vi "Main.vi"() -> ()   [LabVIEW 2015]
doc: "This template is for the Queued Message Handler design pattern.\n\nThe Event Handling Loop generates messages based on user interface actions.\n\nThe Message Handling Loop processes messages generated by the Event Handling Loop, or by other messages. The messages are string values, so new messages can be added easily to the Message Cases case structure in the Message Handling Loop. Each message cluster can also provide an optional value for Message Data, which is a variant that can be converted to whatever message-specific data is required."
uses:
  Custom Controls/config.ctl
  <vilib>/MakerHub/LINX/Private/Type Defs/LINX Ref.ctl
  <vilib>/MakerHub/LINX/Private/Type Defs/Platform.ctl
  <vilib>/MakerHub/LINX/Private/Type Defs/Interface.ctl
  <vilib>/MakerHub/LINX/Private/Device/Type Defs/LINX Device Config.ctl
  <vilib>/MakerHub/LINX/Private/Device/Type Defs/TCP Config.ctl
  <vilib>/MakerHub/LINX/Private/Device/Type Defs/Channels.ctl
  <vilib>/MakerHub/LINX/Public/Peripherals/PWM/PWM Set Duty Cycle 1 Chan.vi
  <vilib>/MakerHub/LINX/Public/Peripherals/Digital/Digital Write 1 Chan.vi
  <vilib>/MakerHub/LINX/Public/Peripherals/Analog/Analog Read 1 Chan.vi
  <vilib>/MakerHub/LINX/Public/Peripherals/Digital/Digital Write N Chans.vi
  <vilib>/MakerHub/LINX/Public/Peripherals/Analog/Analog Read N Chans.vi
  <vilib>/MakerHub/LINX/Private/Local IO/LinxDigitalWrite.vi
  <vilib>/MakerHub/LINX/Public/Utilities/Check Channel.vi
  <vilib>/MakerHub/LINX/Private/Local IO/LinxAnalogRead.vi
  support/Message Queue/Enqueue Message (Single).vi
  <vilib>/Utility/error.llb/Error Cluster From Error Code.vi
  <vilib>/MakerHub/LINX/Public/Utilities/Open Serial.vi
  <vilib>/MakerHub/LINX/Public/Peripherals/PWM/PWM Set Duty Cycle N Chans.vi
  <vilib>/MakerHub/LINX/Private/Utilties/Generate Error.vi
  <vilib>/MakerHub/LINX/Public/Sensors/Motion/Servo/Servo Open One Channel.vi
  <vilib>/MakerHub/LINX/Public/Sensors/Motion/Servo/Servo Set Pulse Width One Channel.vi
  <vilib>/MakerHub/LINX/Public/Sensors/Motion/Servo/Servo Close One Channel.vi
  <vilib>/ErrorRing/Error Ring.xnode
  support/Message Queue/Message Queue.lvlib
  support/User Event - Stop/User Event - Stop.lvlib
  <vilib>/MakerHub/LINX/LMH-LINX.lvlib
  <vilib>/MakerHub/LINX/Public/Sensors/Pmods/GPS/PmodGPS.lvlib
  <vilib>/MakerHub/LINX/Public/Sensors/Motion/Servo/Servo.lvlib
  <vilib>/MakerHub/LINX/Private/Device/Device.lvlib
panel:
  out "Bearing Diff. (deg)":dbl
  out "Actuator Duty Cycle":cluster{"Active":dbl, "Rest":dbl}(graph)
  out "Active Actuator Time (s)":dbl
  out "Required Delay":dbl
  in  "Actuator Channels":T1={"PWM Channel"=9, "Extend Channel"=11, "Retract Channel"=13}
  out "error (out)":errorcluster
  out "Current Bearing (deg)":dbl caption="Numeric"
  out "\"deg\"":string="               deg" caption="String"
  out "Compass":cluster{dbl, dbl}(knob)={0.0, 64.08711650949901} scale=0.0..360.0
  out "Action Feed":string
  out "\"mph\"":string="               mph" caption="String"
  out "Speed Dec":dbl caption="Numeric" format="%#_3g"
  out "\"rpm\"":string="                  rpm" caption="String"
  out "RPM Dec":dbl caption="Numeric"
  out "Steering Angle":dbl(knob) scale=-30.0..30.0
  out "Fuel Meter":dbl(knob) scale=0.0..100.0
  out "Waypoints remaining:":i32 caption="Numeric"
  out "En Route to Waypoint:":i32 caption="Numeric"
  out "Progress Bar":u8(slide) scale=0.0..100.0
  out "Speed Gauge":dbl(knob) scale=0.0..25.0
  out "RPM Gauge":dbl(knob) scale=0.0..7.0
  out "Radio Signal Strength":dbl[](graph)
  out "Steering Angle":T2(graph)
  in  "VISA resource":refnum<visa-resource-name>="COM6"
  out "GPS Data":T3
  in  "WebBrowser":refnum<k7>(container)
  in  "EARTHLib.IApplicationGE 2":refnum<k7>
  out "Init. Panel":cluster{"Boolean":bool, "String":string}[][](array[cluster])
  in  "Abort":bool
  in  "Config":T4
  in  "Open Path":bool caption="Open"
  in  "Start":bool
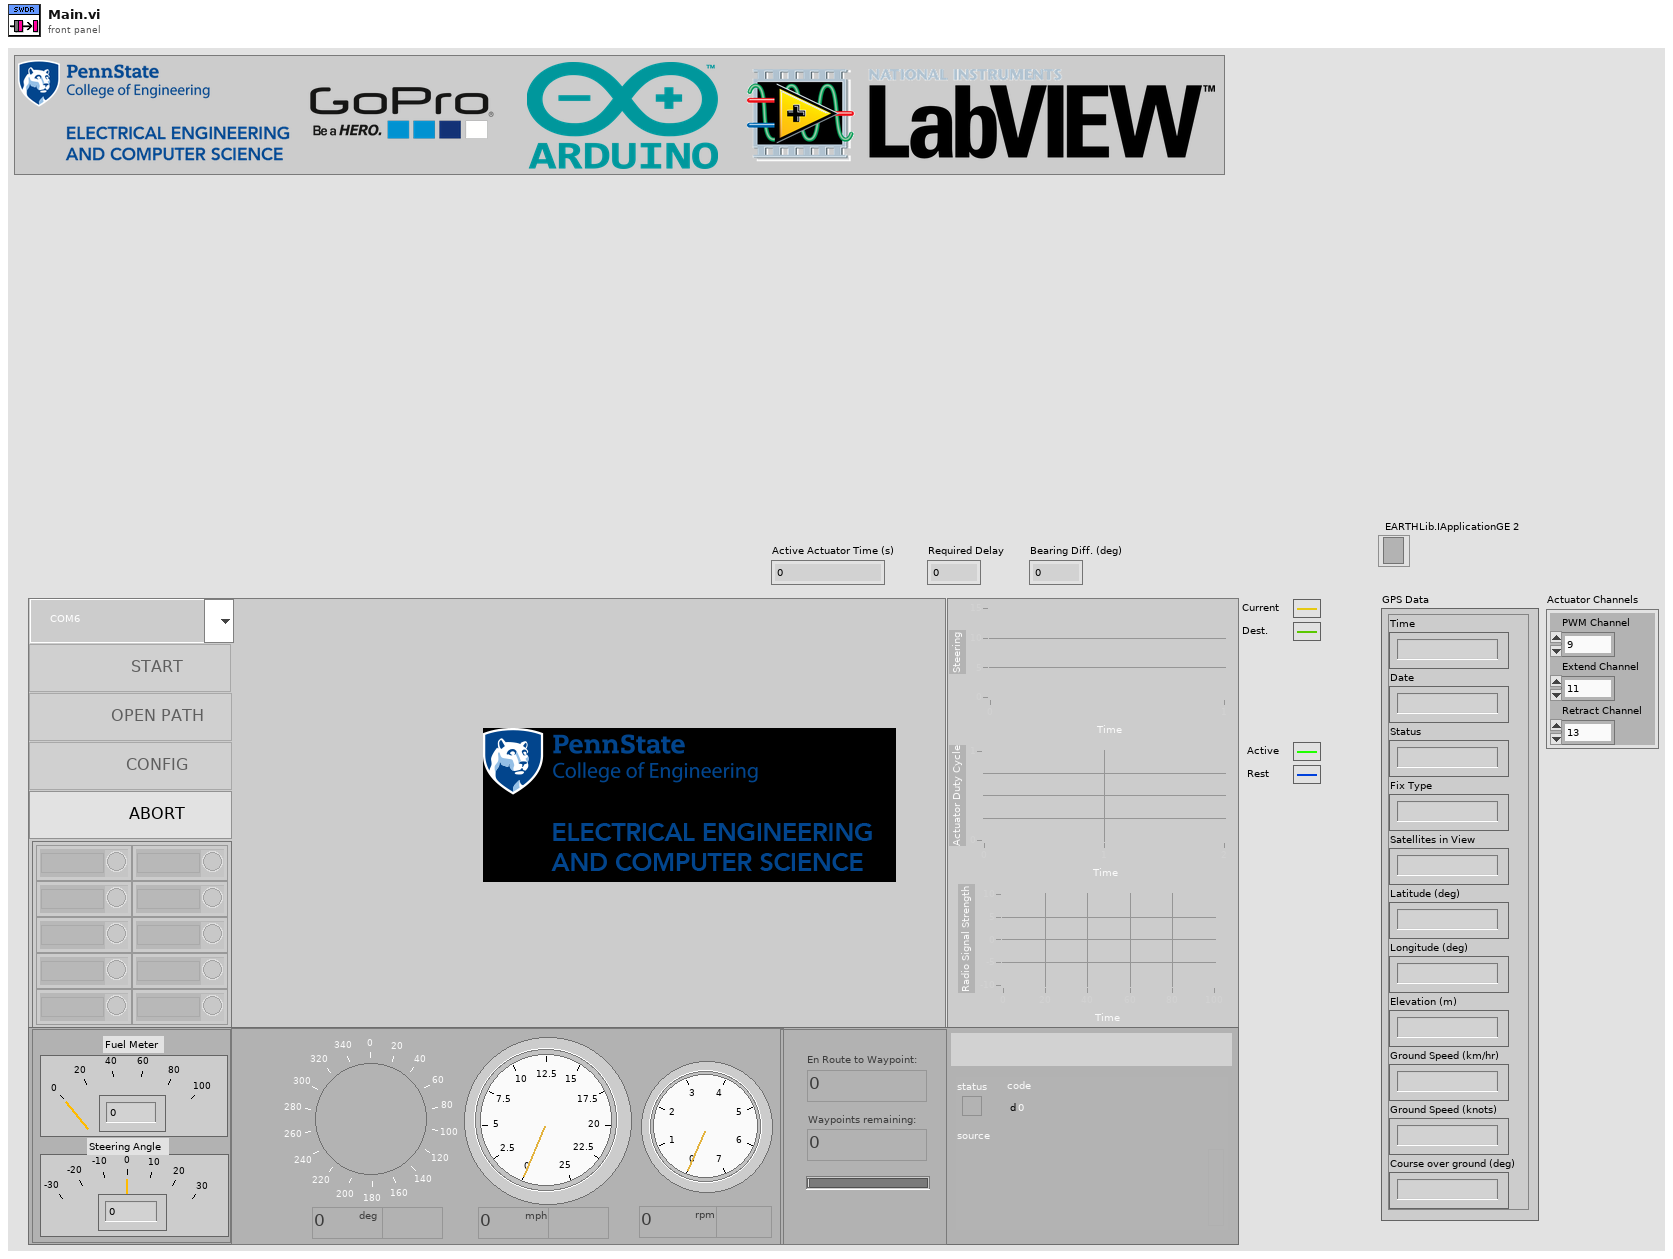
[diagram p1: front panel]
types:
  T1 = cluster{"PWM Channel":u8, "Extend Channel":u8, "Retract Channel":u8}
  T2 = cluster{"Current Bearing (deg)":dbl, "Bearing to Waypoint (deg)":dbl}
  T3 = cluster{"Time":string, "Date":string, "Status":string, "Fix Type":string, "Satellites in View":string, "Latitude (deg)":string, "Longitude (deg)":string, "Elevation (m)":string, "Ground Speed (km/hr)":string, "Ground Speed (knots)":string, "Course over ground (deg)":string}
  T4 = typedef "config.ctl" = bool
  T5 = typedef "LMH-LINX.lvlib/LINX Ref.ctl" = cluster{"IO":T6, "Interface":T7, "LINX Device Config":T8}
  T6 = typedef "LMH-LINX.lvlib/Platform.ctl" = enum16{"Remote", "Local"}
  T7 = typedef "LMH-LINX.lvlib/Interface.ctl" = enum16{"Serial", "TCP"}
  T8 = typedef "LMH-LINX.lvlib/Device.lvlib/LINX Device Config.ctl" = cluster{"Interface":T7, "COM Port":refnum<visa-resource-name>, "TCP Configuration":T9, "Device Family":u8, "Device ID":u8, "Device Name":string, "TCP Ref":refnum<k5>, "Channels":T10}
  T9 = typedef "LMH-LINX.lvlib/Device.lvlib/TCP Config.ctl" = cluster{"IP Address":string, "Port":u16}
  T10 = typedef "LMH-LINX.lvlib/Channels.ctl" = cluster{"DI":u8[], "DO":u8[], "AI":u8[], "AO":u8[], "PWM":u8[], "QE":u8[], "UART":u8[], "I2C 2":u8[], "SPI":u8[], "CAN":u8[], "Servo":u8[], "AI Ref (V)":dbl, "AI Resolution (Bits)":u8, "AO Ref (V)":dbl, "AO Resolution (Bits)":u8}
  T11 = cluster{"Waypoint Array":cluster{"Latitude":dbl, "Longitude":dbl}[], "GPS Data":cluster{"Time":string, "Date":string, "Status":string, "Fix Type":string, "Satellites in View":string, "Latitude (deg)":string, "Longitude (deg)":string, "Elevation (m)":string, "Ground Speed (km/hr)":string, "Ground Speed (knots)":string, "Course over ground (deg)":string}, cluster{"Marker":string, "Path":string, "Markers Coordinates":string[][]}, "LINX Resource":T5, "Google Earth Ref":refnum<k7>, "Time":timestamp, "Waypoint Array Size":i32}
  T12 = typedef "Message Queue.lvlib/All Message Queues.ctl" = cluster{"UI":refnum<queue>}
  T13 = cluster{"Current Bearing":dbl, "Bearing to WP.":dbl}
  T14 = enum8{"Enabled", "Disabled", "Disabled and Grayed Out"}
  T15 = cluster{"Waypoint Array":cluster{"Latitude":dbl, "Longitude":dbl}[], "GPS Data":cluster{"Time":string, "Date":string, "Status":string, "Fix Type":string, "Satellites in View":string, "Latitude (deg)":string, "Longitude (deg)":string, "Elevation (m)":string, "Ground Speed (km/hr)":string, "Ground Speed (knots)":string, "Course over ground (deg)":string}, "Cluster":cluster{"Marker":string, "Path":string, "Markers Coordinates":string[][]}, "LINX Resource":T5, "Google Earth Ref":refnum<k7>, "Time":timestamp, "Waypoint Array Size":i32}
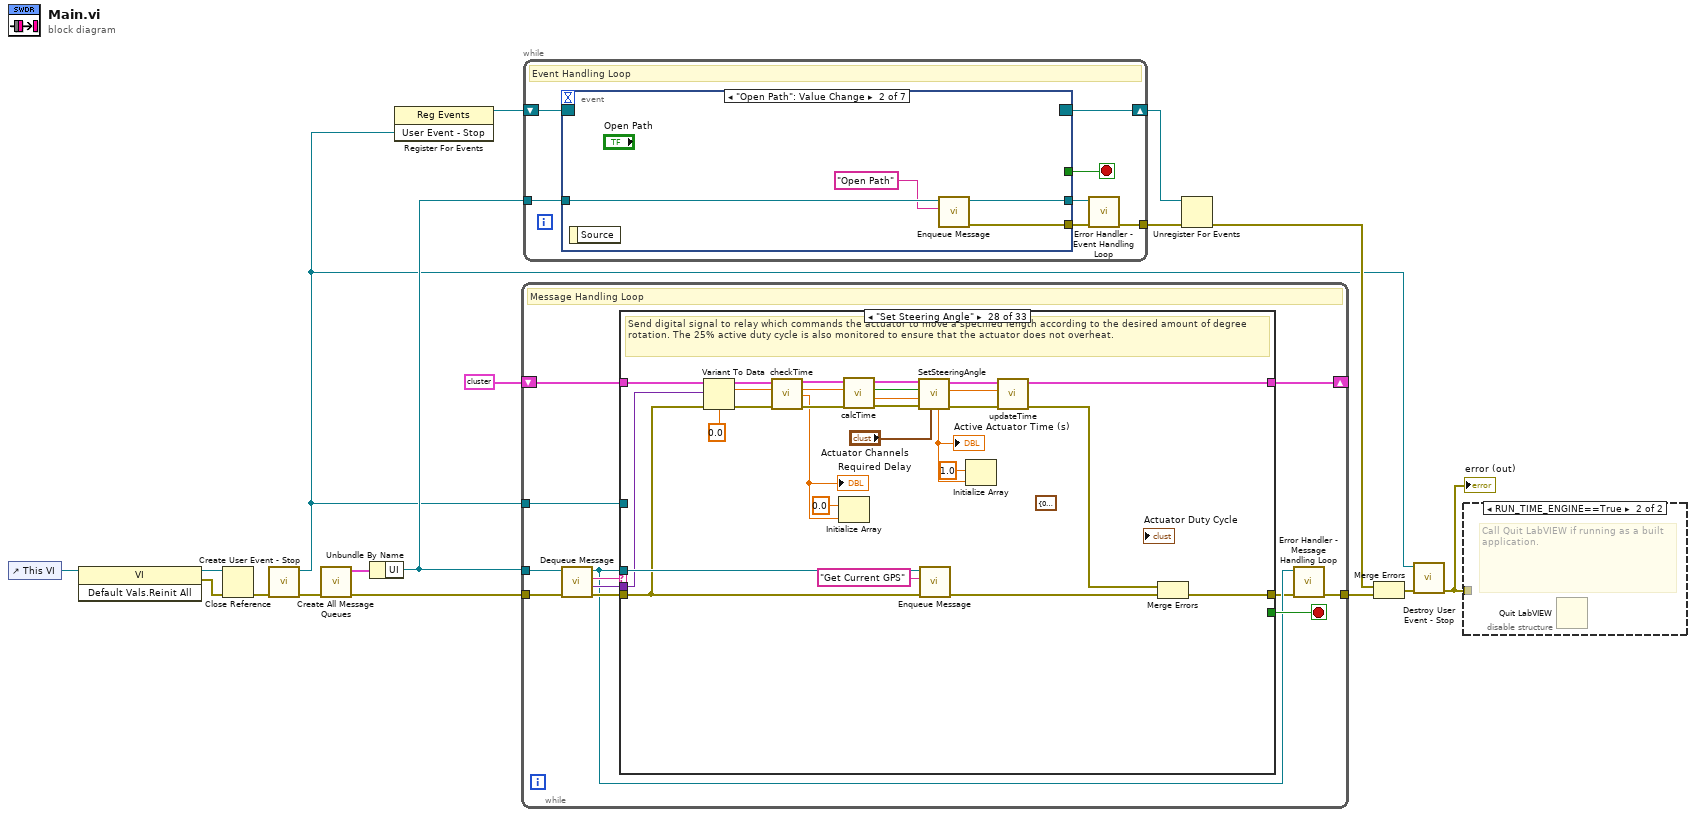
[diagram p0: block diagram]
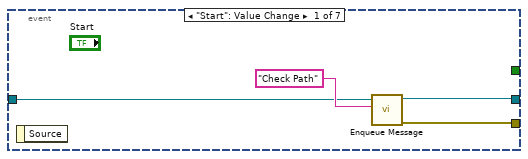
[diagram p3: hidden frame]
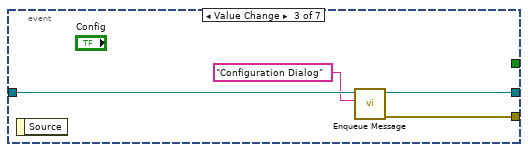
[diagram p4: hidden frame]
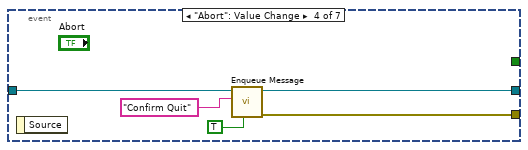
[diagram p5: hidden frame]
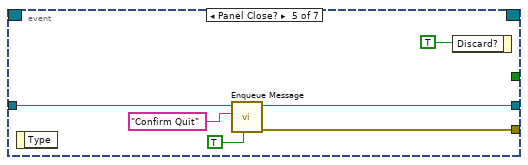
[diagram p6: hidden frame]
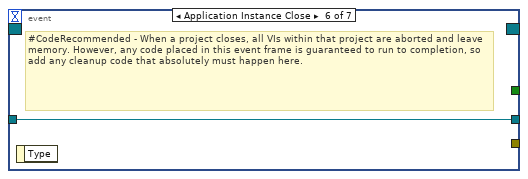
[diagram p7: hidden frame]
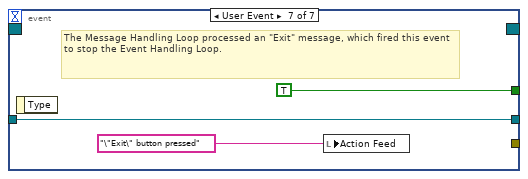
[diagram p8: hidden frame]
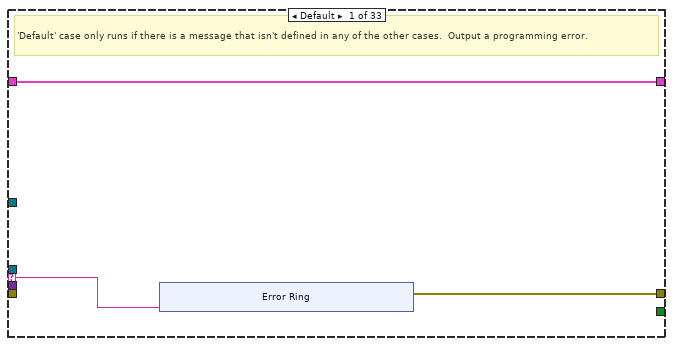
[diagram p9: hidden frame]
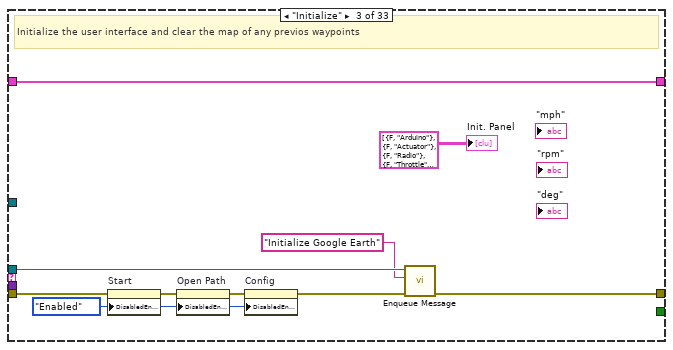
[diagram p11: hidden frame]
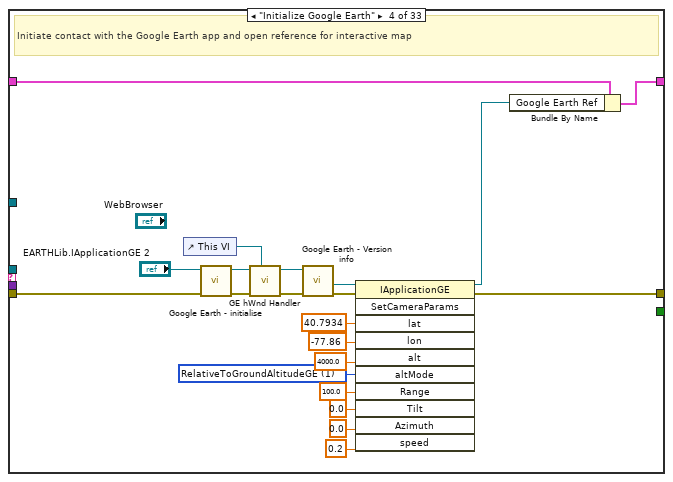
[diagram p12: hidden frame]
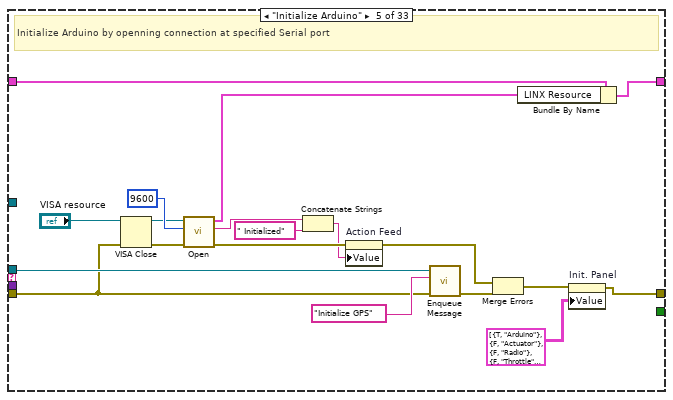
[diagram p13: hidden frame]
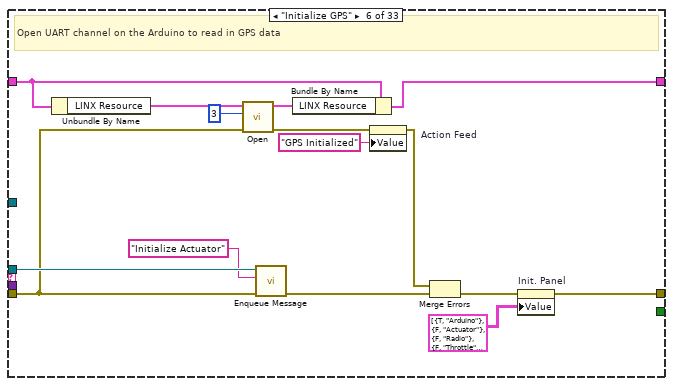
[diagram p14: hidden frame]
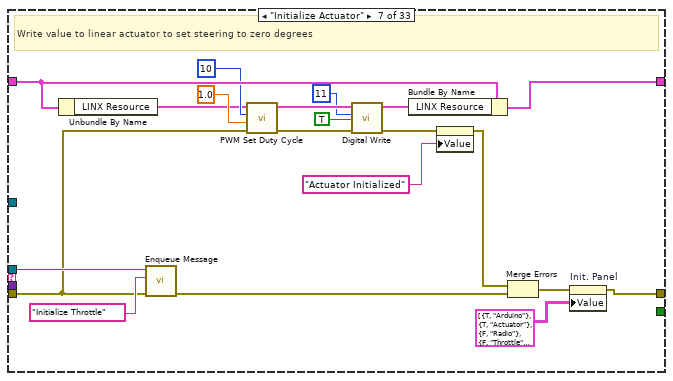
[diagram p15: hidden frame]
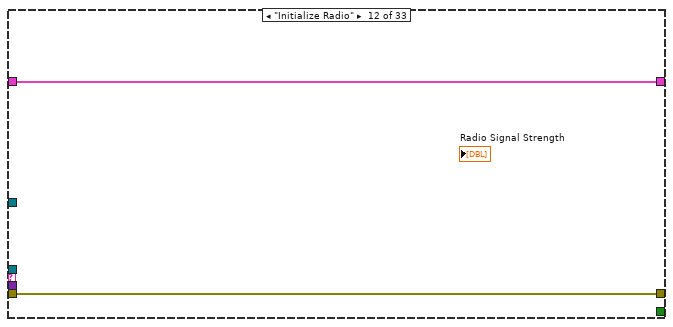
[diagram p20: hidden frame]
diagram:
  n1 = control-ref of="This VI"() -> (w7:refnum<vi>)
  n2 = invoke class="VI" method="Default Vals.Reinit All"(reference=w7) -> (reference out=w6:refnum<vi>, error out=w5:errorcluster)  [unwired: 2 in, 1 out]
  n3 = Close Reference(reference=w6, error in (no error)=w5) -> (error out=w4:errorcluster)
  n4 = call "Create User Event - Stop.vi"("error in (no error)"=w4) -> ("error out"=w14:errorcluster, "User Event - Stop"=w8:refnum<user-event>)  [unwired: 9 in]
  n5 = call "Create All Message Queues.vi"("error in (no error)"=w14) -> ("error out"=w3:errorcluster, "Message Queues out"=w17:T12)  [unwired: 9 in]
  n6 = Unbundle By Name(w17) -> ("UI"=w15:refnum<queue>)
  n7 = register-events(w8) -> (reference out=w9:refnum<event-registration>)  [unwired: 2 in, 1 out]
  n8 = while {
    tunnel: w15 -> [w23]
    tunnel: w8 -> [w28]
    tunnel: w3 -> [w27]
    tunnel: [w21] -> w16
    shift-right: [w18] -> _
    shift-left: T11 {"Waypoint Array"=[], "GPS Data"={"Time"="", "Date"="", "Status"="", "Fix Type"="", "Satellites in View"="", "Latitude (deg)"="", "Longitude (deg)"="", "Elevation (m)"="", "Ground Speed (km/hr)"="", "Ground Speed (knots)"="", "Course over ground (deg)"=""}, {"Marker"="", "Path"="", "Markers Coordinates"=[]}, "LINX Resource"={"IO"=enum."Remote", "Interface"=enum."Serial", "LINX Device Config"={"Interface"=enum."Serial", "COM Port"="", "TCP Configuration"={"IP Address"="", "Port"=0}, "Device Family"=0, "Device ID"=0, "Device Name"="", "TCP Ref"=refnum, "Channels"={"DI"=[], "DO"=[], "AI"=[], "AO"=[], "PWM"=[], "QE"=[], "UART"=[], "I2C 2"=[], "SPI"=[], "CAN"=[], "Servo"=[], "AI Ref (V)"=0.0, "AI Resolution (Bits)"=0, "AO Ref (V)"=0.0, "AO Resolution (Bits)"=0}}}, "Google Earth Ref"=refnum, "Time"=timestamp(0 s since 1904-01-01), "Waypoint Array Size"=0} -> [w19]
    stop <- w29 stop-if-true
    # "Message Handling Loop"
    n9 = call "Dequeue Message.vi"("error in (no error)"=w27, "Message Queue"=w23) -> ("error out"=w26:errorcluster, "Message Data"=w24:variant, "Message"=w25:string, "dup Message Queue"=w22:refnum<queue>)  [unwired: 6 in]
    n10 = case "Message Cases" shown="\"Set Steering Angle\"" w25 {
      selector: w25 -> [w31 _ _ _ _ _ _ _ _ _ _ _ _ _ _ _ _ _ _ _ _ _ _ _ _ _ _ _ _ _ _ _ _]
      tunnel: w22 -> [_ _ w51 _ w89 w102 w122 _ _ _ _ _ w151 _ _ w192 w214 w231 w260 w271 _ _ _ w311 w344 w358 w381 w414 _ _ w435 w456 w469]
      tunnel: w26 -> [_ w41 w45 w66 w87 w99 w108 w127 w129 w131 w133 w135 w148 w162 w173 w183 w215 w230 w255 w270 w297 w299 w301 w312 w342 w360 w372 w404 w421 w429 w437 w453 w463]
      tunnel: [w32 w41 w50 w64 w77 w96 w118 w127 w129 w131 w133 w135 w143 w163 w174 w189 w210 w229 w261 w267 w297 w299 w301 w308 w341 w359 w378 w411 w422 w424 w436 w454 w466] -> w20
      tunnel: [_ _ _ _ _ _ _ _ _ _ _ _ _ _ _ _ _ _ _ _ _ _ _ _ _ _ _ _ _ _ _ _ TRUE] -> w29
      tunnel: w24 -> [_ _ _ _ _ _ _ _ _ _ _ _ _ _ w171 _ _ _ _ _ _ _ _ _ _ _ _ w405 w420 w428 _ _ w460]
      tunnel: w28 -> [_ _ _ _ _ _ _ _ _ _ _ _ _ _ _ _ _ _ _ _ _ _ _ _ _ _ _ _ _ _ _ _ w465]
      tunnel: w19 -> [w30 w40 w47 w55 w75 w92 w117 w126 w128 w130 w132 w134 w137 w168 w179 w187 w208 w227 w253 w266 w296 w298 w300 w305 w325 w355 w368 w406 w416 w423 w430 w445 w459]
      tunnel: [w30 w40 w47 w53 w73 w93 w116 w126 w128 w130 w132 w134 w136 w167 w177 w185 w206 w227 w253 w265 w296 w298 w300 w304 w323 w353 w367 w407 w416 w423 w430 w445 w459] -> w18
      frame Default {
        # "'Default' case only runs if there is a message that isn't defined in any of the other cases.  Output a programming error."
        n11 = xnode "Error Ring"("parameter 0"=w31) -> ("error out"=w32:errorcluster)
      }
      frame "Configure Dialog" {
        # "ideas for configure/settings\n-speed limit\n-tolerance of waypoints\n-driver pins for arduino (maybe an image?)"
        # "Displays dialog so that the user can enter configuration values"
      }
      frame "Initialize" {
        w43 = T14."Enabled" ("Disabled")
        # "Initialize the user interface and clear the map of any previos waypoints"
        n12 = property on="Start" class="Bool"(error in=w45, "DisabledEnum"=w43) -> (error out=w42:errorcluster)  [unwired: 1 in, 1 out]
        n13 = property on="Open Path" class="Bool"(error in=w42, "DisabledEnum"=w43) -> (error out=w46:errorcluster)  [unwired: 1 in, 1 out]
        n14 = property on="Config" class="Bool"(error in=w46, "DisabledEnum"=w43) -> (error out=w44:errorcluster)  [unwired: 1 in, 1 out]
        n15 = call-poly "Enqueue Message.vi"("error in (no error)"=w44, "Message"="Initialize Google Earth", "Message Queue"=w51) -> ("error out"=w50:errorcluster)  [unwired: 7 in, 1 out]
        "Init. Panel" <- cluster{"Boolean 10":bool, "String":string}[][] [[{"Boolean 10"=FALSE, "String"="Arduino"}, {"Boolean 10"=FALSE, "String"="Actuator"}], [{"Boolean 10"=FALSE, "String"="Radio"}, {"Boolean 10"=FALSE, "String"="Throttle"}], [{"Boolean 10"=FALSE, "String"="GPS"}, {"Boolean 10"=FALSE, "String"="RPI3"}], [{"Boolean 10"=FALSE, "String"="Speed G."}, {"Boolean 10"=FALSE, "String"="Camera"}], [{"Boolean 10"=FALSE, "String"="Gas G."}, {"Boolean 10"=FALSE, "String"="Path"}]] ("Array")
      }
      frame "Initialize Google Earth" {
        w60 = 1 items=["RelativeToGroundAltitudeGE"=1, "AbsoluteAltitudeGE"=2] ("altMode")
        # "Initiate contact with the Google Earth app and open reference for interactive map"
        n16 = control-ref of="This VI"() -> (w71:refnum<vi>)
        n17 = call "Google Earth - initialise.vi"("error in (no error)"=w66, "EARTHLib.IApplicationGE"="EARTHLib.IApplicationGE 2") -> ("error out"=w68:errorcluster, "Refnum Out"=w72:refnum<k7>)  [unwired: 7 in, 1 out]
        n18 = call "GE hWnd Handler.vi"("This VI"=w71, "error in"=w68, "Refnum In"=w72) -> ("error out"=w67:errorcluster, "Refnum Out"=w70:refnum<k7>)  [unwired: 7 in]
        n19 = call "Google Earth - Version info.vi"("error in"=w67, "Refnum In"=w70) -> ("error out"=w65:errorcluster, "Refnum Out"=w52:refnum<k7>)  [unwired: 4 in, 4 out]
        n20 = invoke class="IApplicationGE" method="SetCameraParams"(reference=w52, error in=w65, "lat"=40.7934, "lon"=-77.86, "alt"=4000.0, "altMode"=w60, "Range"=100.0, "Tilt"=0.0, "Azimuth"=0.0, "speed"=0.2) -> (reference out=w54:refnum<k7>, error out=w64:errorcluster)  [unwired: 1 in, 9 out]
        n21 = Bundle By Name(cluster=w55, "Google Earth Ref"=w54) -> (w53:T11)
      }
      frame "Initialize Arduino" {
        # "Initialize Arduino by openning connection at specified Serial port"
        n22 = VISA Close(VISA resource name="VISA resource", error in (no error)=w87) -> (error out=w86:errorcluster)
        n23 = call-poly <vilib>:"Open.vi"("Error In"=w86, "Baud Rate Override"=u32 9600, "Serial Port"="VISA resource") -> ("Error Out"=w84:errorcluster, "Device Name"=w82:string, "LINX Resource"=w74:T5)  [unwired: 6 in]
        n24 = Concatenate Strings(w82, " Initialized" ("string")) -> (w81:string)
        n25 = property on="Action Feed" class="Str"(error in=w84, "Value"=w81) -> (error out=w83:errorcluster)  [unwired: 1 in, 1 out]
        n26 = call-poly "Enqueue Message.vi"("error in (no error)"=w87, "Message"="Initialize GPS", "Message Queue"=w89) -> ("error out"=w85:errorcluster)  [unwired: 7 in, 1 out]
        n27 = Merge Errors(w83, w85) -> (w78:errorcluster)
        n28 = Bundle By Name(cluster=w75, "LINX Resource"=w74) -> (w73:T11)
        n29 = property on="Init. Panel" class="Arr (strict)"(error in=w78, "Value"=cluster{"Boolean 10":bool, "String":string}[][] [[{"Boolean 10"=TRUE, "String"="Arduino"}, {"Boolean 10"=FALSE, "String"="Actuator"}], [{"Boolean 10"=FALSE, "String"="Radio"}, {"Boolean 10"=FALSE, "String"="Throttle"}], [{"Boolean 10"=FALSE, "String"="GPS"}, {"Boolean 10"=FALSE, "String"="RPI3"}], [{"Boolean 10"=FALSE, "String"="Speed G."}, {"Boolean 10"=FALSE, "String"="Camera"}], [{"Boolean 10"=FALSE, "String"="Gas G."}, {"Boolean 10"=TRUE, "String"="Path"}]] ("Array")) -> (error out=w77:errorcluster)  [unwired: 1 in, 1 out]
      }
      frame "Initialize GPS" {
        # "Open UART channel on the Arduino to read in GPS data"
        n30 = Unbundle By Name(w92) -> ("LINX Resource"=w91:T5)
        n31 = call <vilib>:"Open.vi"("Error In"=w99, "UART Channel (0)"=u8 3, "LINX Ref"=w91) -> ("Error Out"=w105:errorcluster, "LINX Resource"=w94:T5)  [unwired: 7 in]
        n32 = call-poly "Enqueue Message.vi"("error in (no error)"=w99, "Message"="Initialize Actuator", "Message Queue"=w102) -> ("error out"=w101:errorcluster)  [unwired: 7 in, 1 out]
        n33 = Bundle By Name(cluster=w92, "LINX Resource"=w94) -> (w93:T11)
        n34 = property on="Action Feed" class="Str"(error in=w105, "Value"="GPS Initialized" ("Action Feed")) -> (error out=w103:errorcluster)  [unwired: 1 in, 1 out]
        n35 = Merge Errors(w103, w101) -> (w97:errorcluster)
        n36 = property on="Init. Panel" class="Arr (strict)"(error in=w97, "Value"=cluster{"Boolean 10":bool, "String":string}[][] [[{"Boolean 10"=TRUE, "String"="Arduino"}, {"Boolean 10"=FALSE, "String"="Actuator"}], [{"Boolean 10"=FALSE, "String"="Radio"}, {"Boolean 10"=FALSE, "String"="Throttle"}], [{"Boolean 10"=TRUE, "String"="GPS"}, {"Boolean 10"=FALSE, "String"="RPI3"}], [{"Boolean 10"=FALSE, "String"="Speed G."}, {"Boolean 10"=FALSE, "String"="Camera"}], [{"Boolean 10"=FALSE, "String"="Gas G."}, {"Boolean 10"=TRUE, "String"="Path"}]] ("Array")) -> (error out=w96:errorcluster)  [unwired: 1 in, 1 out]
      }
      frame "Initialize Actuator" {
        # "Write value to linear actuator to set steering to zero degrees"
        n37 = Unbundle By Name(w117) -> ("LINX Resource"=w111:T5)
        n38 = call-poly "Enqueue Message.vi"("error in (no error)"=w108, "Message"="Initialize Throttle", "Message Queue"=w122) -> ("error out"=w121:errorcluster)  [unwired: 7 in, 1 out]
        n39 = call-poly <vilib>:"PWM Set Duty Cycle.vi"("Error In"=w108, "Duty Cycle (0-1)"=1.0, "PWM Channel"=u8 10, "LINX Resource"=w111) -> ("Error Out"=w114:errorcluster, "LINX Resource"=w115:T5)  [unwired: 6 in]
        n40 = call-poly <vilib>:"Digital Write.vi"("Error In"=w114, "Output Value"=TRUE, "DO Channel"=u8 11, "LINX Resource"=w115) -> ("Error Out"=w107:errorcluster, "LINX Resource"=w106:T5)  [unwired: 6 in]
        n41 = Bundle By Name(cluster=w117, "LINX Resource"=w106) -> (w116:T11)
        n42 = property on="Action Feed" class="Str"(error in=w107, "Value"="Actuator Initialized" ("Action Feed")) -> (error out=w124:errorcluster)  [unwired: 1 in, 1 out]
        n43 = Merge Errors(w124, w121) -> (w119:errorcluster)
        n44 = property on="Init. Panel" class="Arr (strict)"(error in=w119, "Value"=cluster{"Boolean 10":bool, "String":string}[][] [[{"Boolean 10"=TRUE, "String"="Arduino"}, {"Boolean 10"=TRUE, "String"="Actuator"}], [{"Boolean 10"=FALSE, "String"="Radio"}, {"Boolean 10"=FALSE, "String"="Throttle"}], [{"Boolean 10"=TRUE, "String"="GPS"}, {"Boolean 10"=FALSE, "String"="RPI3"}], [{"Boolean 10"=FALSE, "String"="Speed G."}, {"Boolean 10"=FALSE, "String"="Camera"}], [{"Boolean 10"=FALSE, "String"="Gas G."}, {"Boolean 10"=TRUE, "String"="Path"}]] ("Array")) -> (error out=w118:errorcluster)  [unwired: 1 in, 1 out]
      }
      frame "Initialize Gas Gauge" {
        # "Read initial value from the gas tank sensor to ensure that sensor is functioning properly."
      }
      frame "Initialize RPI Feed" {
      }
      frame "Initialize Camera" {
      }
      frame "Initialize Speed Gauge" {
      }
      frame "Initialize Radio" {
      }
      frame "Initialize Throttle" {
        w146 = u8 2 ("Servo Channel")
        # "Set throttle to value of zero, which disengages it at startup"
        n45 = Unbundle By Name(w137) -> ("LINX Resource"=w141:T5)
        n46 = call-poly <vilib>:"Servo Open.vi"("Error In"=w148, "Servo Channel"=w146, "LINX Resource"=w141) -> ("Error Out"=w149:errorcluster, "LINX Resource"=w150:T5)  [unwired: 7 in]
        n47 = for {
          N: 100 -> [_]
          shift-right: [w158] -> w147
          shift-left: w149 -> [w159]
          tunnel: w146 -> [w157]
          shift-right: [w155] -> w138
          shift-left: w150 -> [w160]
          n48 = call-poly <vilib>:"Servo Set Pulse Width.vi"("Error In"=w159, "Pulse Width (uS)"=u16 200, "Servo Channel"=w157, "LINX Resource"=w160) -> ("Error Out"=w158:errorcluster, "LINX Resource"=w155:T5)  [unwired: 6 in]
          n49 = Wait (ms)(milliseconds to wait=u32 0) -> ()  [unwired: 1 out]
        }
        n50 = property on="Action Feed" class="Str"(error in=w147, "Value"="Throttle Initialized" ("Action Feed")) -> (error out=w139:errorcluster)  [unwired: 1 in, 1 out]
        n51 = Bundle By Name(cluster=w137, "LINX Resource"=w138) -> (w136:T11)
        n52 = call-poly "Enqueue Message.vi"("error in (no error)"=w148, "Message"="Accelerate Throttle", "Message Queue"=w151) -> ("error out"=w140:errorcluster)  [unwired: 7 in, 1 out]
        n53 = Merge Errors(w139, w140) -> (w144:errorcluster)
        n54 = property on="Init. Panel" class="Arr (strict)"(error in=w144, "Value"=cluster{"Boolean 10":bool, "String":string}[][] [[{"Boolean 10"=TRUE, "String"="Arduino"}, {"Boolean 10"=TRUE, "String"="Actuator"}], [{"Boolean 10"=FALSE, "String"="Radio"}, {"Boolean 10"=TRUE, "String"="Throttle"}], [{"Boolean 10"=TRUE, "String"="GPS"}, {"Boolean 10"=FALSE, "String"="RPI3"}], [{"Boolean 10"=FALSE, "String"="Speed G."}, {"Boolean 10"=FALSE, "String"="Camera"}], [{"Boolean 10"=FALSE, "String"="Gas G."}, {"Boolean 10"=TRUE, "String"="Path"}]] ("Array")) -> (error out=w143:errorcluster)  [unwired: 1 in, 1 out]
      }
      frame "Read Temp" {
        n55 = Unbundle By Name(w168) -> ("LINX Resource"=w166:T5)
        n56 = call-poly <vilib>:"Analog Read.vi"("Error In"=w162, "Analog Channel"=u8 0, "LINX Resource"=w166) -> ("Error Out"=w164:errorcluster, "LINX Resource"=w165:T5)  [unwired: 5 in, 2 out]
        n57 = Bundle By Name(cluster=w168, "LINX Resource"=w165) -> (w167:T11)
        n58 = Merge Errors(w164, w162) -> (w163:errorcluster)
      }
      frame "Control Fan" {
        # "Controls the on/off state of the fan in one condition by utilizing the variant messages."
        n59 = Variant To Data(error in=w173, type=FALSE ("Output Value"), Variant=w171) -> (data=w169:bool, error out=w172:errorcluster)
        n60 = Unbundle By Name(w179) -> ("LINX Resource"=w180:T5)
        n61 = call-poly <vilib>:"Digital Write.vi"("Error In"=w172, "Output Value"=w169, "DO Channel"=u8 4, "LINX Resource"=w180) -> ("Error Out"=w175:errorcluster, "LINX Resource"=w178:T5)  [unwired: 6 in]
        n62 = Bundle By Name(cluster=w179, "LINX Resource"=w178) -> (w177:T11)
        n63 = Merge Errors(w175, w172) -> (w174:errorcluster)
      }
      frame "Accelerate Throttle" {
        # "Controlled acceleration of the throttle"
        n64 = Unbundle By Name(w187) -> ("LINX Resource"=w184:T5)
        n65 = property on="Action Feed" class="Str"(error in=w183, "Value"="Accelerating throttle" ("Action Feed")) -> (error out=w182:errorcluster)  [unwired: 1 in, 1 out]
        n66 = while {
          tunnel: u8 2 ("Servo Channel") -> [w205]
          shift-right: [w201] -> w186
          shift-left: w184 -> [w202]
          shift-right: [w200] -> w190
          shift-left: w182 -> [w199]
          i -> [w198]
          stop <- w203 stop-if-true
          n67 = Divide(x=w198, y=85) -> (x/y=w194:dbl)
          "Speed Gauge" <- w194
          "Speed Dec" <- w194
          n68 = call-poly <vilib>:"Servo Set Pulse Width.vi"("Error In"=w199, "Pulse Width (uS)"=w198, "Servo Channel"=w205, "LINX Resource"=w202) -> ("Error Out"=w200:errorcluster, "LINX Resource"=w201:T5)  [unwired: 6 in]
          n69 = Divide(x=w194, y=6.798) -> (x/y=→"RPM Gauge" →"RPM Dec":dbl)
          n70 = Equal?(x=700, y=w198) -> (x = y?=w203:bool)
        }
        n71 = Bundle By Name(cluster=w187, "LINX Resource"=w186) -> (w185:T11)
        n72 = call-poly "Enqueue Message.vi"("error in (no error)"=w183, "Message"="Get Current GPS", "Message Queue"=w192) -> ("error out"=w191:errorcluster)  [unwired: 7 in, 1 out]
        n73 = Merge Errors(w190, w191) -> (w189:errorcluster)
      }
      frame "Decelerate Throttle" {
        # "Controlled deceleration of the throttle"
        n74 = Unbundle By Name(w208) -> ("LINX Resource"=w209:T5)
        n75 = while {
          tunnel: u8 2 ("Servo Channel") -> [w226]
          shift-right: [w224] -> w207
          shift-left: w209 -> [w225]
          shift-right: [w223] -> w211
          shift-left: w215 -> [w222]
          i -> [w219]
          stop <- w217 stop-if-true
          n76 = Subtract(x=1500, y=w219) -> (x-y=w218:i32)
          n77 = Equal To 0?(x=w218) -> (x = 0?=w217:bool)
          n78 = Wait (ms)(milliseconds to wait=u32 20) -> ()  [unwired: 1 out]
          n79 = call-poly <vilib>:"Servo Set Pulse Width.vi"("Error In"=w222, "Pulse Width (uS)"=w218, "Servo Channel"=w226, "LINX Resource"=w225) -> ("Error Out"=w223:errorcluster, "LINX Resource"=w224:T5)  [unwired: 6 in]
        }
        n80 = Bundle By Name(cluster=w208, "LINX Resource"=w207) -> (w206:T11)
        n81 = call-poly "Enqueue Message.vi"("error in (no error)"=w215, "Message"="Exit", "Message Queue"=w214) -> ("error out"=w212:errorcluster)  [unwired: 7 in, 1 out]
        n82 = Merge Errors(w211, w212) -> (w210:errorcluster)
      }
      frame "Check Path" {
        # "Check the waypoint path array to see if it is empty or not then proceed accordingly"
        n83 = Unbundle By Name(w227) -> ("Waypoint Array"=w228:cluster{"Latitude":dbl, "Longitude":dbl}[])
        n84 = Empty Array?(array=w228) -> (empty?=w232:bool)
        n85 = case shown="False" w232 {
          tunnel: w231 -> [w237 w243]
          tunnel: w230 -> [w238 w242]
          tunnel: [w233 w240] -> w229
          frame False {
            # "If there are values in the waypoint in the array then proceed to initialization"
            n86 = call-poly "Enqueue Message.vi"("error in (no error)"=w238, "Message"="Disable Controls", "Message Queue"=w237) -> ("error out"=w234:errorcluster)  [unwired: 7 in, 1 out]
            n87 = property on="Init. Panel" class="Arr (strict)"(error in=w234, "Value"=cluster{"Boolean":bool, "String":string}[][] [[{"Boolean"=FALSE, "String"="Arduino"}, {"Boolean"=FALSE, "String"="Actuator"}], [{"Boolean"=FALSE, "String"="Radio"}, {"Boolean"=FALSE, "String"="Throttle"}], [{"Boolean"=FALSE, "String"="GPS"}, {"Boolean"=FALSE, "String"="RPI3"}], [{"Boolean"=FALSE, "String"="Speed G."}, {"Boolean"=FALSE, "String"="Camera"}], [{"Boolean"=FALSE, "String"="Gas G."}, {"Boolean"=TRUE, "String"="Path"}]] ("Init. Panel")) -> (error out=w233:errorcluster)  [unwired: 1 in, 1 out]
          }
          frame True {
            # "If empty then provide dialog"
            n88 = Two Button Dialog(message="GPS path empty - you must add/open a path before starting. Would you like to launch the GPS add path window now?", 1:"NO" ("F button name (\"Cancel\")"), 2:"YES" ("T button name (\"OK\")")) -> (T button?=w244:bool)
            n89 = case shown="True" w244 {
              tunnel: w243 -> [_ w252]
              tunnel: w242 -> [w248 w250]
              tunnel: [w248 w249] -> w241
              frame False {
              }
              frame True {
                n90 = call-poly "Enqueue Message.vi"("error in (no error)"=w250, "Message"="Open Path", "Message Queue"=w252) -> ("error out"=w249:errorcluster)  [unwired: 7 in, 1 out]
              }
            }
            n91 = property on="Init. Panel" class="Arr (strict)"(error in=w241, "Value"=cluster{"Boolean":bool, "String":string}[][] [[{"Boolean"=FALSE, "String"="Arduino"}, {"Boolean"=FALSE, "String"="Actuator"}], [{"Boolean"=FALSE, "String"="Radio"}, {"Boolean"=FALSE, "String"="Throttle"}], [{"Boolean"=FALSE, "String"="GPS"}, {"Boolean"=FALSE, "String"="RPI3"}], [{"Boolean"=FALSE, "String"="Speed G."}, {"Boolean"=FALSE, "String"="Camera"}], [{"Boolean"=FALSE, "String"="Gas G."}, {"Boolean"=FALSE, "String"="Path"}]] ("Init. Panel")) -> (error out=w240:errorcluster)  [unwired: 1 in, 1 out]
          }
        }
      }
      frame "Disable Controls" {
        w257 = T14."Disabled and Grayed Out" ("Disabled")
        # "Disable front panel controls so that the user does not re-initiate the start sequence"
        n92 = property on="Start" class="Bool"(error in=w255, "DisabledEnum"=w257) -> (error out=w256:errorcluster)  [unwired: 1 in, 1 out]
        n93 = property on="Open Path" class="Bool"(error in=w256, "DisabledEnum"=w257) -> (error out=w258:errorcluster)  [unwired: 1 in, 1 out]
        n94 = property on="Config" class="Bool"(error in=w258, "DisabledEnum"=w257) -> (error out=w254:errorcluster)  [unwired: 1 in, 1 out]
        n95 = call-poly "Enqueue Message.vi"("error in (no error)"=w254, "Message"="Initialize Arduino", "Message Queue"=w260) -> ("error out"=w261:errorcluster)  [unwired: 7 in, 1 out]
      }
      frame "Open Path" {
        # "Open a path that has been saved to an Excel File"
        n96 = call "File Dialog"("error in"=w270) -> ("selected path"=w269:path, "cancelled"=w262:bool, "error out"=w268:errorcluster)  [unwired: 6 in, 6 out]
        n97 = case shown="False" w262 {
          tunnel: w271 -> [w286 w292]
          tunnel: w270 -> [w284 w294]
          tunnel: w269 -> [w283 _]
          tunnel: w268 -> [w282 w289]
          tunnel: w266 -> [w277 w295]
          tunnel: [w276 w295] -> w265
          tunnel: [w275 w293] -> w264
          tunnel: [w274 w288] -> w263
          frame False {
            n98 = call "ParseKML.vi"("error (in)"=w282, ".kml File Path"=w283) -> ("error (out)"=w274:errorcluster, "Waypoint Array"=w273:cluster{"Latitude":dbl, "Longitude":dbl}[])  [unwired: 8 in]
            n99 = Empty Array?(array=w273) -> (empty?=w281:bool)
            n100 = Select(t="error processing .kml file", s=w281, f=".kml file successfully read" ("Message")) -> (s? t:f=w278:string)
            n101 = Array Size(array=w273) -> (size(s)=w272:i32)
            n102 = call-poly "Enqueue Message.vi"("error in (no error)"=w284, "Message Data"=w278, "Message"="Update Display", "Message Queue"=w286) -> ("error out"=w275:errorcluster)  [unwired: 6 in, 1 out]
            n103 = Bundle By Name(cluster=w277, "Waypoint Array"=w273, "Waypoint Array Size"=w272) -> (w276:T11)
          }
          frame True {
            # "clear the file cancellation error \nso that the program is not terminated\nby the error"
            n104 = call <vilib>:"Clear Errors.vi"("error in (no error)"=w289, "specific error code to clear (0: all)"=43) -> ("error out"=w288:errorcluster)  [unwired: 4 in, 1 out]
            n105 = call-poly "Enqueue Message.vi"("error in (no error)"=w294, "Message Data"="File openning cancelled" ("Message"), "Message"="Update Display", "Message Queue"=w292) -> ("error out"=w293:errorcluster)  [unwired: 6 in, 1 out]
          }
        }
        n106 = Merge Errors(w263, w264) -> (w267:errorcluster)
      }
      frame "Check Speed" {
      }
      frame "Check Gas" {
      }
      frame "Check Camera" {
        # "Checks the incoming Raspberry Pi 3 serial feed to see if there is any detected obstacle that must be avoided"
      }
      frame "Get Current GPS" {
        # "Get current GPS location to be used by steering module"
        n107 = Unbundle By Name(w305) -> ("LINX Resource"=w306:T5)
        n108 = while {
          shift-right: [w315] -> w309
          shift-left: w312 -> [w320]
          shift-right: [w318] -> w302
          shift-left: w306 -> [w322]
          tunnel: [w314] -> w303
          stop <- w313 continue-if-true
          n109 = call <vilib>:"Read.vi"("Error In"=w320, "UART Channel (0)"=u8 3, "LINX Resource"=w322) -> ("Error Out"=w316:errorcluster, "GPS Data"=w317:T3, "LINX Resource"=w319:T5)  [unwired: 6 in]
          "GPS Data" <- w317
          n110 = call "LatLongEmpty"("error (in)"=w316, "GPS Data"=w317, "LINX Resource"=w319) -> ("error (out)"=w315:errorcluster, "Empty or not in range?"=w313:bool, "GPS Data"=w314:T3, "LINX Resource"=w318:T5)  [unwired: 5 in]
        }
        n111 = call-poly "Enqueue Message.vi"("error in (no error)"=w312, "Message"="Show Current Location", "Message Queue"=w311) -> ("error out"=w310:errorcluster)  [unwired: 7 in, 1 out]
        n112 = Bundle By Name(cluster=w305, "LINX Resource"=w302, "GPS Data"=w303) -> (w304:T11)
        n113 = Merge Errors(w309, w310) -> (w308:errorcluster)
      }
      frame "Show Current Location" {
        w339 = 1 items=["RelativeToGroundAltitudeGE"=1, "AbsoluteAltitudeGE"=2] ("altMode")
        # "Shows the current location of the snowdrone on Google Earth by writing a custom .kml file and reading it."
        n114 = Unbundle By Name(w325) -> ("Google Earth Ref"=w326:refnum<k7>, "GPS Data.Latitude (deg)"=w328:string, "GPS Data.Longitude (deg)"=w327:string)
        n115 = Fract/Exp String To Number(string=w327) -> (number=w346:dbl)  [unwired: 3 in, 1 out]
        n116 = Negate(x=w346) -> (-x=w330:dbl)
        n117 = Number To Fractional String(number=w330) -> (F-format string=w345:string)  [unwired: 3 in]
        n118 = call "WriteKML.vi"("Latitude"=w328, "Longitude"=w345) -> ("Path"=w348:string)  [unwired: 6 in]
        n119 = invoke class="IApplicationGE" method="OpenKmlFile"(reference=w326, error in=w342, "fileName"=w348, "suppressMessages"=0) -> (reference out=w334:refnum<k7>, error out=w333:errorcluster)  [unwired: 1 in, 3 out]
        n120 = Fract/Exp String To Number(string=w328) -> (number=w329:dbl)  [unwired: 3 in, 1 out]
        n121 = call-poly "Enqueue Message.vi"("error in (no error)"=w342, "Message"="Check Location", "Message Queue"=w344) -> ("error out"=w331:errorcluster)  [unwired: 7 in, 1 out]
        n122 = invoke class="IApplicationGE" method="SetCameraParams"(reference=w334, error in=w333, "lat"=w329, "lon"=w330, "alt"=4000.0, "altMode"=w339, "Range"=100.0, "Tilt"=0.0, "Azimuth"=0.0, "speed"=0.2) -> (reference out=w324:refnum<k7>, error out=w332:errorcluster)  [unwired: 1 in, 9 out]
        n123 = Bundle By Name(cluster=w325, "Google Earth Ref"=w324) -> (w323:T11)
        n124 = Merge Errors(w332, w331) -> (w341:errorcluster)
      }
      frame "Check Location" {
        # "Check the current location to see if the waypoint has been reached or not"
        n125 = Unbundle By Name(w355) -> ("Waypoint Array Size"=w349:i32, "Waypoint Array"=w357:cluster{"Latitude":dbl, "Longitude":dbl}[], "GPS Data"=w356:T3)
        n126 = call "CheckLocation.vi"("Message Queue"=w358, "Waypoint Array Size"=w349, "Waypoint Array (in)"=w357, "GPS Data"=w356, "error (in)"=w360) -> ("Waypoint Array (out)"=w354:cluster{"Latitude":dbl, "Longitude":dbl}[], "En Route"=→"En Route to Waypoint:":i32, "Waypoints remaining"=→"Waypoints remaining:":i32, "Progress Bar"=→"Progress Bar":u8, "error (out)"=w359:errorcluster)  [unwired: 6 in]
        n127 = Bundle By Name(cluster=w355, "Waypoint Array"=w354) -> (w353:T11)
      }
      frame "Get Steering Angle" {
        (unwired) "Get Current GPS" ("Message")
        # "Send digital output command to control the relay connected to the actuator"
        n128 = Unbundle By Name(w368) -> ("Waypoint Array"=w376:cluster{"Latitude":dbl, "Longitude":dbl}[], "GPS Data"=w375:T3, "LINX Resource"=w371:T5)
        n129 = while {
          shift-right: [w384] -> w370
          shift-left: w372 -> [w389]
          shift-right: [w387] -> w366
          shift-left: w371 -> [w391]
          tunnel: [w383] -> w369
          stop <- w382 continue-if-true
          n130 = call <vilib>:"Read.vi"("Error In"=w389, "UART Channel (0)"=u8 3, "LINX Resource"=w391) -> ("Error Out"=w385:errorcluster, "GPS Data"=w386:T3, "LINX Resource"=w388:T5)  [unwired: 6 in]
          n131 = call "LatLongEmpty"("error (in)"=w385, "GPS Data"=w386, "LINX Resource"=w388) -> ("error (out)"=w384:errorcluster, "Empty or not in range?"=w382:bool, "GPS Data"=w383:T3, "LINX Resource"=w387:T5)  [unwired: 5 in]
        }
        n132 = call "ComputeSteeringAngle.vi"("error (in)"=w370, "Current GPS Data"=w369, "Previous GPS Data"=w375, "Waypoint Array"=w376) -> ("error (out)"=w379:errorcluster, "Steering Angle"=w377:dbl, "Bearing to Waypoint (deg)"=w364:dbl, "Current Bearing (deg)"=w365:dbl, "Bearing Diff. (deg)"=→"Bearing Diff. (deg)":dbl)  [unwired: 3 in]
        "Steering Angle" <- w377
        "Current Bearing (deg)" <- w365
        n133 = Bundle By Name(cluster=T13 {"Current Bearing"=0.0, "Bearing to WP."=0.0} ("Compass"), "Current Bearing"=w365, "Bearing to WP."=w364) -> (→"Compass":T13)
        n134 = Bundle("Current Bearing (deg)"=w365, "Bearing to Waypoint (deg)"=w364) -> (→"Steering Angle":T2)  [unwired: 1 in]
        n135 = Bundle By Name(cluster=w368, "LINX Resource"=w366) -> (w367:T11)
        n136 = call-poly "Enqueue Message.vi"("error in (no error)"=w372, "Message Data"=w377, "Message"="Set Steering Angle", "Message Queue"=w381) -> ("error out"=w380:errorcluster)  [unwired: 6 in, 1 out]
        n137 = Merge Errors(w379, w380) -> (w378:errorcluster)
      }
      frame "Set Steering Angle" {
        (unwired) cluster{"Active":dbl, "Rest":dbl} {"Active"=0.0, "Rest"=0.0}
        # "Send digital signal to relay which commands the actuator to move a specified length according to the desired amount of degree rotation. The 25% active duty cycle is also monitored to ensure that the actuator does not overheat."
        n138 = Variant To Data(error in=w404, type=0.0 ("Steering Angle"), Variant=w405) -> (data=w401:dbl, error out=w403:errorcluster)
        n139 = call "checkTime.vi"("error (in)"=w403, "Data (in)"=w406) -> ("error (out)"=w397:errorcluster, "Required Delay"=w395:dbl, "Data (out)"=w402:T15)  [unwired: 7 in]
        "Required Delay" <- w395
        n140 = Initialize Array(0.0 ("element"), w395) -> ()  [unwired: 1 out]
        n141 = call "calcTime.vi"("error in (no error)"=w397, "Steering Angle"=w401) -> ("error (out)"=w399:errorcluster, "Active Actuator Time"=w393:dbl, "Positive Angle?"=w400:bool)  [unwired: 7 in]
        "Active Actuator Time (s)" <- w393
        n142 = call "SetSteeringAngle.vi"("Actuator Channels"="Actuator Channels", "error (in)"=w399, "Actuator Active Time"=w393, "Positive?"=w400, "Data (in)"=w402) -> ("error (out)"=w410:errorcluster, "Actuator Active Time (out)"=w396:dbl, "Data (out)"=w408:T15)  [unwired: 4 in]
        n143 = call-poly "Enqueue Message.vi"("error in (no error)"=w404, "Message"="Get Current GPS", "Message Queue"=w414) -> ("error out"=w412:errorcluster)  [unwired: 7 in, 1 out]
        n144 = Initialize Array(1.0 ("element"), w393) -> ()  [unwired: 1 out]
        n145 = call "updateTime.vi"("error in (no error)"=w410, "Actuator Active Time"=w396, "Data (in)"=w408) -> ("error out"=w409:errorcluster, "Data (out)"=w407:T15)  [unwired: 7 in]
        n146 = Merge Errors(w409, w412) -> (w411:errorcluster)
      }
      frame "Update Display" {
        # "Update Display - Convert the message data to a string to display in the Data Display indicator."
        n147 = Variant To Data(error in=w421, type="", Variant=w420) -> (data=→"Action Feed":string, error out=w418:errorcluster)
        n148 = Merge Errors(w418) -> (w422:errorcluster)
      }
      frame "Error" {
        # "Error - Display an error dialog. This message is sent by the \"Error Handler\" VIs at the end of other loops in this application."
        n149 = Variant To Data(error in=w429, type=errorcluster {"status"=FALSE, "code"=0, "source"=""} ("error constant"), Variant=w428) -> (data=w426:errorcluster, error out=w425:errorcluster)
        n150 = call <vilib>:"Simple Error Handler.vi"("error in (no error)"=w426) -> ()  [unwired: 4 in, 5 out]
        n151 = Merge Errors(w425) -> (w424:errorcluster)
      }
      frame "Confirm Quit" {
        # "Confirm Quit - Message that can confirm whether or not the user wants to exit the application."
        n152 = Two Button Dialog(message="Are you sure that you want to abort the sequence?", 1:"NO" ("F button name (\"Cancel\")"), 2:"YES" ("T button name (\"OK\")")) -> (T button?=w431:bool)
        n153 = case shown="True" w431 {
          tunnel: w437 -> [w438 w444]
          tunnel: [w438 w443] -> w436
          tunnel: w435 -> [_ w441]
          frame False {
          }
          frame True {
            n154 = call-poly "Enqueue Message.vi"("Priority Message? (F)"=TRUE, "error in (no error)"=w444, "Message"="Close Resource", "Message Queue"=w441) -> ("error out"=w442:errorcluster)  [unwired: 6 in, 1 out]
            n155 = Merge Errors(w442) -> (w443:errorcluster)
          }
        }
      }
      frame "Close Resource" {
        # "Close resouce to Arduino and all ports that were previously opened"
        n156 = Unbundle By Name(w445) -> ("LINX Resource"=w446:T5)
        n157 = call <vilib>:"Close.vi"("error in (no error)"=w453, "UART Channel (0)"=u8 3, "LINX Resource"=w446) -> ("error out"=w451:errorcluster, "LINX Resource out"=w452:T5)  [unwired: 7 in]
        n158 = call-poly <vilib>:"Servo Close.vi"("Error In"=w451, "Servo Channel"=u8 2, "LINX Resource"=w452) -> ("Error Out"=w448:errorcluster, "LINX Resource"=w449:T5)  [unwired: 7 in]
        n159 = call <vilib>:"Close.vi"("Error In"=w448, "LINX Resource"=w449) -> ("Error Out"=w447:errorcluster)  [unwired: 9 in]
        n160 = Merge Errors(w447, w453) -> (w455:errorcluster)
        n161 = call-poly "Enqueue Message.vi"("error in (no error)"=w455, "Message Data"=w455, "Message"="Exit", "Message Queue"=w456) -> ("error out"=w454:errorcluster)  [unwired: 6 in, 1 out]
      }
      frame "Exit" {
        # "Exit - Exit the application."
        n162 = Variant To Data(type=errorcluster {"status"=FALSE, "code"=0, "source"=""} ("error constant"), Variant=w460) -> (data=w461:errorcluster)  [unwired: 1 in, 1 out]
        n163 = call <vilib>:"Simple Error Handler.vi"("error in (no error)"=w461) -> ()  [unwired: 4 in, 5 out]
        n164 = call "Fire User Event - Stop.vi"("User Event - Stop"=w465) -> ("error out"=w464:errorcluster)  [unwired: 10 in]
        n165 = Release Queue(queue=w469, error in (no error)=w463) -> (error out=w467:errorcluster)  [unwired: 1 in, 2 out]
        n166 = Merge Errors(w464, w467) -> (w466:errorcluster)
      }
    }
    n167 = call "Error Handler - Message Handling Loop.vi"("error in (no error)"=w20, "Message Queue"=w22) -> ("dup error in"=w21:errorcluster)  [unwired: 8 in, 1 out]
  }
  n168 = while {
    tunnel: w15 -> [w476]
    shift-right: [w474] -> w11
    shift-left: w9 -> [w475]
    tunnel: [w470] -> w10
    stop <- w472 stop-if-true
    # "Event Handling Loop"
    n169 = event shown="[1] \"Open Path\": Value Change" {
      selector: w475 -> [_ _ _ _ _ _ _]
      dyn-events: [_ _ _ _ _ _ _] -> w474
      timeout: _ -> [_ _ _ _ _ _ _]
      tunnel: [_ _ _ _ _ _ TRUE ("Discard?")] -> w472
      tunnel: w476 -> [w479 w484 w488 w493 w498 w500 w503]
      tunnel: [w477 w483 w486 w492 w497 _ _] -> w473
      tunnel: [w478 w482 w487 w491 w496 w500 w503] -> w471
      event "Start": Value Change {
        n170 = event-data() -> ()  [unwired: 1 in, 1 out]
        n171 = call-poly "Enqueue Message.vi"("Message"="Check Path", "Message Queue"=w479) -> ("error out"=w477:errorcluster, "dup Message Queue"=w478:refnum<queue>)  [unwired: 8 in]
      }
      event "Open Path": Value Change {
        n172 = event-data() -> ()  [unwired: 1 in, 1 out]
        n173 = call-poly "Enqueue Message.vi"("Message"="Open Path", "Message Queue"=w484) -> ("error out"=w483:errorcluster, "dup Message Queue"=w482:refnum<queue>)  [unwired: 8 in]
      }
      event Value Change {
        n174 = event-data() -> ()  [unwired: 1 in, 1 out]
        n175 = call-poly "Enqueue Message.vi"("Message"="Configuration Dialog", "Message Queue"=w488) -> ("error out"=w486:errorcluster, "dup Message Queue"=w487:refnum<queue>)  [unwired: 8 in]
      }
      event "Abort": Value Change {
        n176 = event-data() -> ()  [unwired: 1 in, 1 out]
        n177 = call-poly "Enqueue Message.vi"("Priority Message? (F)"=TRUE, "Message"="Confirm Quit", "Message Queue"=w493) -> ("error out"=w492:errorcluster, "dup Message Queue"=w491:refnum<queue>)  [unwired: 7 in]
      }
      event Panel Close? {
        n178 = event-data() -> ()  [unwired: 1 in, 1 out]
        n179 = call-poly "Enqueue Message.vi"("Priority Message? (F)"=TRUE, "Message"="Confirm Quit", "Message Queue"=w498) -> ("error out"=w497:errorcluster, "dup Message Queue"=w496:refnum<queue>)  [unwired: 7 in]
        n180 = event-data("Discard?"=TRUE) -> ()  [unwired: 1 in, 1 out]
      }
      event Application Instance Close {
        # "#CodeRecommended - When a project closes, all VIs within that project are aborted and leave memory. However, any code placed in this event frame is guaranteed to run to completion, so add any cleanup code that absolutely must happen here."
        n181 = event-data() -> ()  [unwired: 1 in, 1 out]
      }
      event User Event {
        # "The Message Handling Loop processed an \"Exit\" message, which fired this event to stop the Event Handling Loop."
        n182 = event-data() -> ()  [unwired: 1 in, 1 out]
        n183 = local write "Action Feed"("\"Exit\" button pressed" ("VI Stopped")) -> ()
      }
    }
    n184 = call "Error Handler - Event Handling Loop.vi"("error in (no error)"=w473, "Message Queue"=w471) -> ("dup error in"=w470:errorcluster)  [unwired: 8 in, 1 out]
  }
  n185 = Unregister For Events(event registration refnum=w11, error in=w10) -> (error out=w12:errorcluster)
  n186 = Merge Errors(w12, w16) -> (w13:errorcluster)
  n187 = call "Destroy User Event - Stop.vi"("error in (no error)"=w13, "User Event - Stop"=w8) -> ("error out"=w2:errorcluster)  [unwired: 9 in]
  "error (out)" <- w2
  n188 = disable-structure shown="RUN_TIME_ENGINE==True" {
    disable-tunnel: w2 -> [_ _]
    frame condition #0 (active) {
    }
    frame condition #1 {
      # "Call Quit LabVIEW if running as a built application."
      n189 = Quit LabVIEW() -> ()  [unwired: 1 in]
    }
  }
